vi "initializemotors.vi"(9 "MG17Motor Z":refnum<k7>(container), 10 "MG17Motor Y":refnum<k7>(container), 11 "Automation Refnum in":refnum<k7>(container)) -> (2 "Array":errorcluster[](array[cluster]), 3 "Array 2":refnum<k7>[](array[refnum]))   [LabVIEW 2014]
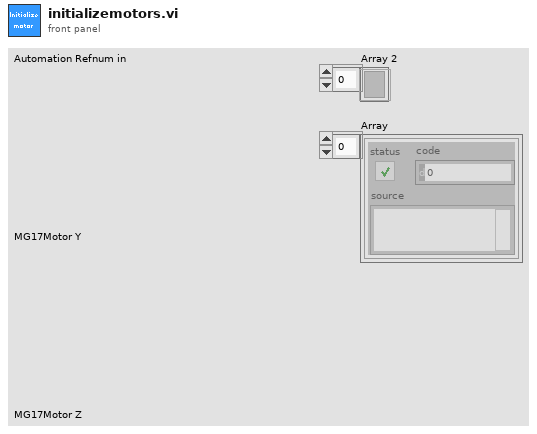
[diagram p1: front panel]
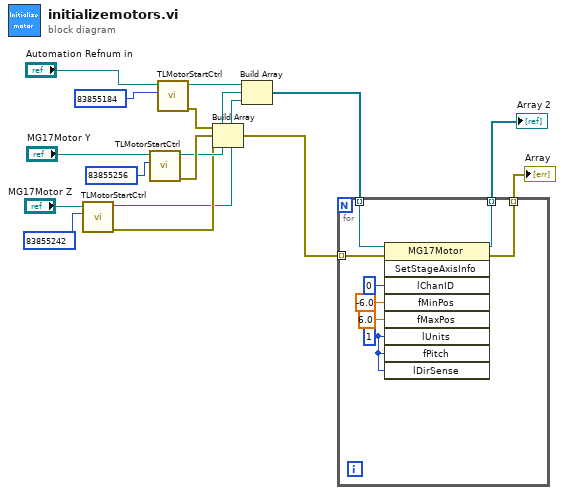
[diagram p0: block diagram]
diagram:
  n1 = call "TLMotorStartCtrl.vi"("SerialNum"=83855242 ("lChanID"), "Motor Ref"="MG17Motor Z") -> ("Error Out"=w2:errorcluster, "Motor Ref"=w1:refnum<k7>)  [unwired: 4 in]
  n2 = call "TLMotorStartCtrl.vi"("SerialNum"=83855256 ("lChanID"), "Motor Ref"="MG17Motor Y") -> ("Error Out"=w16:errorcluster, "Motor Ref"=w14:refnum<k7>)  [unwired: 4 in]
  n3 = call "TLMotorStartCtrl.vi"("SerialNum"=83855184 ("lChanID"), "Motor Ref"="Automation Refnum in") -> ("Error Out"=w15:errorcluster, "Motor Ref"=w13:refnum<k7>)  [unwired: 4 in]
  n4 = Build Array(w15, w16, w2) -> (w5:errorcluster[])
  n5 = Build Array(w13, w14, w1) -> (w6:refnum<k7>[])
  n6 = for {
    tunnel: w6 -> [w24] mode=indexing
    tunnel: w5 -> [w23] mode=indexing
    tunnel: [w22] -> w4 mode=indexing
    tunnel: [w21] -> w3 mode=indexing
    w17 = 1 ("lUnits")
    n7 = invoke class="MG17Motor" method="SetStageAxisInfo"(reference=w24, error in=w23, "lChanID"=0, "fMinPos"=sgl -6.0, "fMaxPos"=sgl 6.0, "lUnits"=w17, "fPitch"=w17, "lDirSense"=w17) -> (reference out=w21:refnum<k7>, error out=w22:errorcluster)  [unwired: 1 in, 7 out]
  }
  "Array" <- w4
  "Array 2" <- w3
